vi "局部变量的使用.vi"() -> ()   [LabVIEW 2018]
panel:
  out "字符串 2":string
  in  "确定按钮":bool
  in  "字符串":string
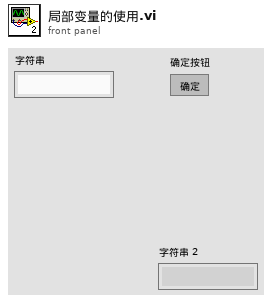
[diagram p1: front panel]
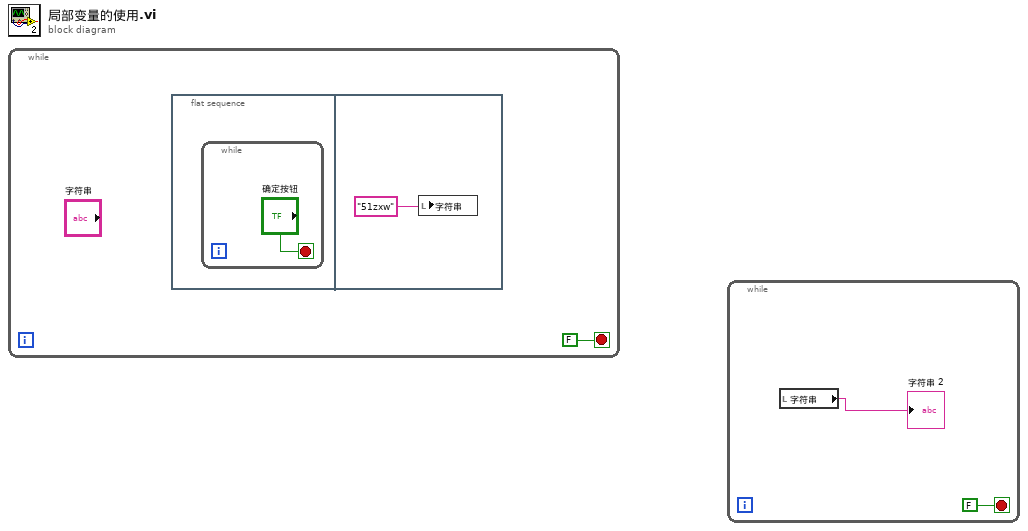
[diagram p0: block diagram]
diagram:
  n1 = while {
    stop <- FALSE stop-if-true
    n2 = flat-sequence {
      frame #0 {
        n3 = while {
          stop <- "确定按钮" stop-if-true
        }
      }
      frame #1 {
        n4 = local write "字符串"("51zxw") -> ()
      }
    }
  }
  n5 = while {
    stop <- FALSE stop-if-true
    n6 = local read "字符串"() -> (→"字符串 2":string)
  }
